vi "high_field_probe.vi"() -> ()   [LabVIEW 2011]
uses:
  <vilib>/Analysis/NI_AALBase.lvlib
panel:
  out "normalized amplitude":dbl
  out "average power":dbl
  in  "Center Freq":dbl=1000.0
  in  "threshold":dbl=0.001
  in  "rate":dbl=20000.0
  in  "number of samples":i32=500
  out "data":dynamicdata(graph)
  out "Waveform Chart":dbl(graph)
  out "amplitude":dbl
  out "frequency":dbl
  in  "stop":bool
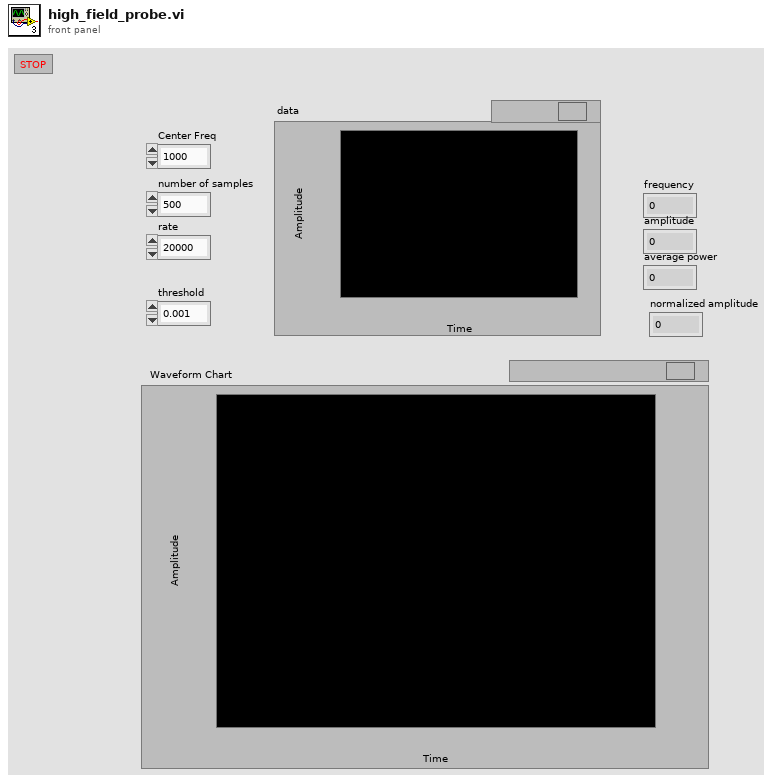
[diagram p1: front panel]
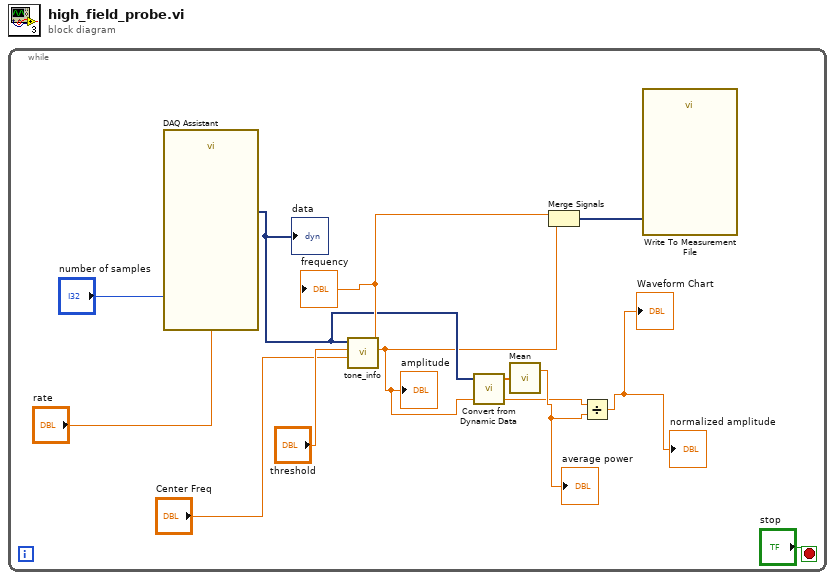
[diagram p0: block diagram]
diagram:
  n1 = while {
    stop <- "stop" stop-if-true
    n2 = call "DAQ Assistant"("rate"="rate", "number of samples"="number of samples") -> ("data"=w4:dynamicdata)  [unwired: 15 in, 2 out]
    "data" <- w4
    n3 = call "tone_info.vi"("Center Freq"="Center Freq", "threshold"="threshold", "time signal in"=w4) -> ("amplitude"=w2:dbl, "frequency"=w8:dbl)  [unwired: 6 in, 1 out]
    "frequency" <- w8
    "amplitude" <- w2
    n4 = call "Convert from Dynamic Data"("Dynamic Data Type"=w4) -> ("Array"=w5:dbl[])  [unwired: 3 in]
    n5 = call <vilib>:"Mean.vi"("X"=w5) -> ("mean"=w3:dbl)  [unwired: 1 out]
    "average power" <- w3
    n6 = Merge Signals(w8, w2) -> (w7:dynamicdata)
    n7 = Divide(x=w2, y=w3) -> (x/y=→"Waveform Chart" →"normalized amplitude":dbl)
    n8 = call "Write To Measurement File"("Signals"=w7) -> ()  [unwired: 16 in, 3 out]
  }
